vi "ziExample-Module-Scope.vi"() -> ()   [LabVIEW 2009]
doc: "Control a Zurich instrument device via the LabOne Labview API. \nRequirements: Zurich Instruments MFLI, HF2 or UHFLI \nThis example shows how to start a scope module and retrieve data.\n\n© Zurich Instruments AG, www.zhinst.com"
uses:
  <instrlib>/Zurich Instruments LabOne/Public/Modules/ziTypeModEnum.ctl
  <instrlib>/Zurich Instruments LabOne/Public/Configure/ziSetValueDouble.vi
  <instrlib>/Zurich Instruments LabOne/Public/Modules/ziModSetValueDoubleArray.vi
  <instrlib>/Zurich Instruments LabOne/Public/Configure/ziGetValueString.vi
  <instrlib>/Zurich Instruments LabOne/Public/Configure/ziSetValueDoubleArray.vi
  <instrlib>/Zurich Instruments LabOne/Public/Modules/ziModGetScopeWave.vi
  <instrlib>/Zurich Instruments LabOne/Public/Modules/ziModSetValueDouble.vi
  <instrlib>/Zurich Instruments LabOne/Zurich Instruments LabOne.lvlib
panel:
  in  "method":u16(ring)=1 items=["Exponential", "Uniform"]
  in  "length":i32=100 caption="Length (pts)"
  in  "segmentedcount":i32=100 caption="segmented count"
  in  "segmented":bool=TRUE
  out "?":sgl[][](graph)
  in  "mode":u16(ring)=1 items=["Time Domain"=1, "Freq Domain FFT"=3]
  in  "stop":bool
  in  "averagerweight":dbl=1.0 caption="averager/weight"
  out "?":cluster{dbl[], "Data Float":sgl[]}[](graph)
  out "Error Out":errorcluster
  in  "Address":string="DEV"
  out "Selected Device":string
  in  "subscribepath":string="scopes/0/wave" caption="Subscribe Path"
  # "Only for non-HF2"
  # "ziExample-Module-Scope.vi\nRequirements: HF2LI, UHFLI or MFLI\nsee block diagram for VI description"
  # "Tested Devices:\n- HF2LI\n- UHFLI\n- MFLI"
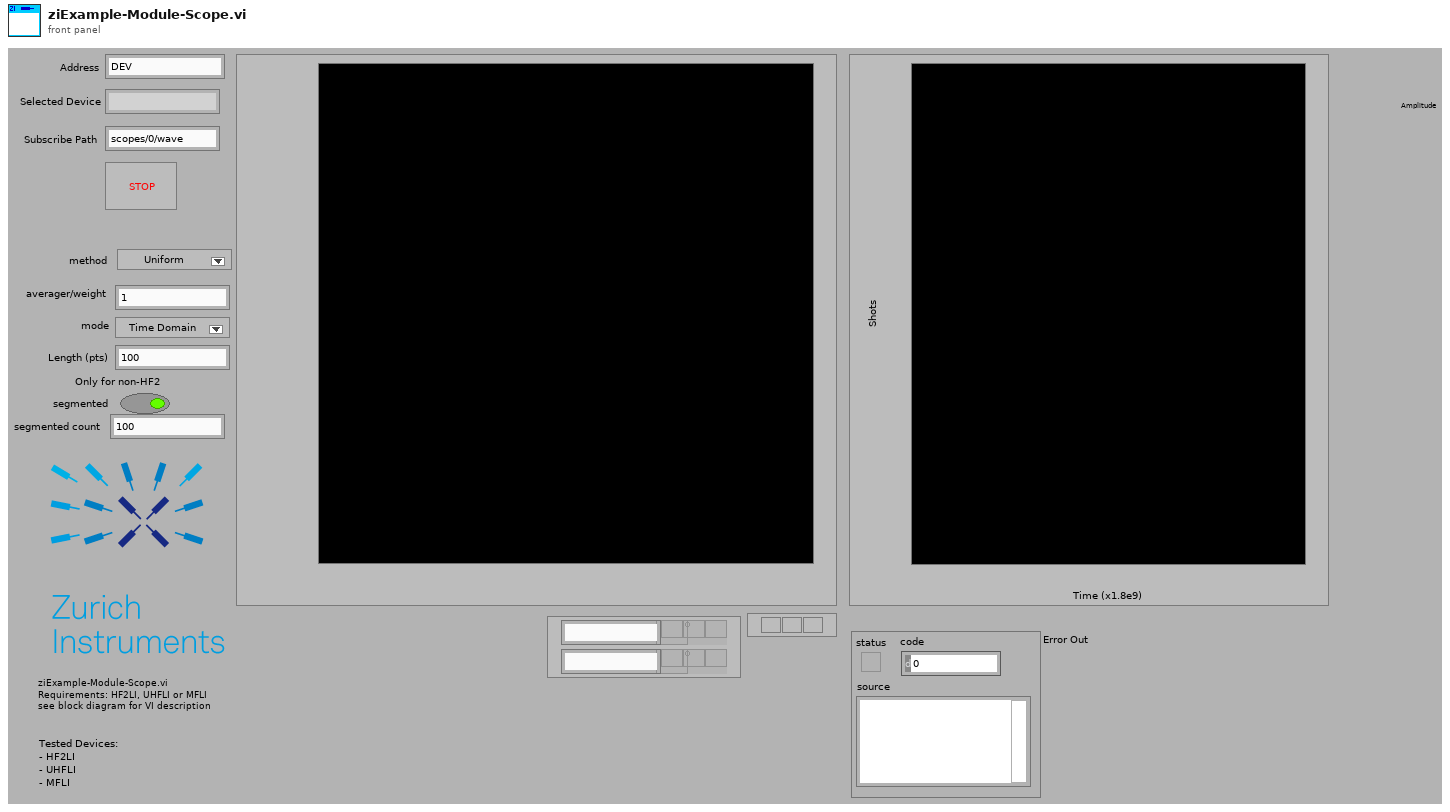
[diagram p1: front panel]
types:
  T1 = typedef "Zurich Instruments LabOne.lvlib/ziTypeModEnum.ctl" = u16
  T2 = typedef "Zurich Instruments LabOne.lvlib/ziTypeHandle.ctl" = cluster{"handleValid":bool, "Conn":u64, "Path Prefix":string, "Handle":u64, "Connected":bool, "Clockbase(s)":dbl}
  T3 = typedef "Zurich Instruments LabOne.lvlib/ziTypeModHandle.ctl" = cluster{"handleValid":bool, "Conn":u64, "ModHandle":u64, "moduleID":string, "Path Prefix":string}
  T4 = typedef "Zurich Instruments LabOne.lvlib/ziTypeModResults.ctl" = cluster{"PathArray":string[], "ValueType":T5, "NoOfResults":u64, "ziGenericHeader":T6[]}
  T5 = typedef "Zurich Instruments LabOne.lvlib/ziTypePollType.ctl" = enum16{"NONE", "DOUBLE_DATA", "INTEGER_DATA", "DEMOD_SAMPLE", "SCOPE_WAVE_HF2", "AUXIN_SAMPLE", "DIO_SAMPLE", "BYTE_ARRAY", "PWA_WAVE", "9", "10", "11", "12", "13", "14", "15", "TREE_CHANGE_DEPRI", "17", "ERROR", "19", "20", "21", "22", "23", "24", "25", "26", "27", "28", "29", "30", "31", "DOUBLE_DATA_TS", "INTEGER_DATA_TS", "34", "SCOPE_WAVE", "SCOPE_WAVE_EX", "37", "BYTE_ARRAY_TS", "39", "40", "41", "42", "43", "44", "45", "CNT_DATA", "47", "TREE_CHANGE", "49", "50", "51", "52", "53", "54", "55", "56", "57", "58", "59", "60", "61", "62", "63", "SWEEPER_DATA", "SPECTRUM_DATA", "ADVISOR_DATA", "VECTOR_DATA", "IMP_DATA", "SHF_GENERATOR_WAVEFORM_DATA", "SHF_RESULT_LOGGER_DATA", "SHF_SCOPE_DATA", "DEMOD_VECTOR"}
  T6 = typedef "Zurich Instruments LabOne.lvlib/ziTypeModGenericHeader.ctl" = cluster{"HeaderType":enum8{"HEADER_TYPE_NONE", "HEADER_TYPE_SWTRIGGER", "HEADER_TYPE_SWEEPER"}, "SampleFormat":u8, "SystemTime":timestamp, "CreatedTimeStamp":u64, "ChangedTimeStamp":u64, "Flags":u32, "ChunkSizeBytes":u64, "Name":string, "Status":u32, "GroupIndex":u32, "Color":u32, "ActiveRow":u32, "TriggerNumber":u64, "GridRows":u32, "GridCols":u32, "GridMode":u32, "GridOperation":u32, "GridDirection":u32, "GridRepetitions":u32, "GridColDelta":dbl, "GridColOffset":dbl, "GridRowDelta":dbl, "GridRowOffset":dbl, "Bandwidth":dbl, "Center":dbl, "Nenbw":dbl}
  T7 = typedef "Zurich Instruments LabOne.lvlib/ziTypeScopeWaveGrid.ctl" = cluster{"Timestamp (ticks)":u64, "Timestamp Trigger (ticks)":u64, "dt (s)":dbl, "Channel Enable":u8[], "Channel Input":enum8{"Signal Input 1", "Signal Input 2", "Trigger Input 1", "Trigger Input 2", "Aux Output 1", "Aux Output 2", "Aux Output 3", "Aux Output 4", "Aux Input 1", "Aux Input 2"}[], "Trigger Enable":u64, "Trigger Input":u64, "Channel BW Limit":u8[], "Channel Math":u8[], "Channel Scaling":sgl[], "Sequence Number":u32, "Segment Number":u32, "Block Number":u32, "Data Transfer Mode":enum8{"Single Transfer", "Block Transfer", "Continuous Transfer", "FFT Single Transfer"}, "Block Marker":enum8{"None", "End of Block"}, "Flags":u8, "Sample Format":enum8{"Int16", "Int32", "Float32", "reserved", "Int16 Interleaved", "Int32 Interleaved", "Float32 Interleaved"}, "Sample Count":u32, "Channel Offset":dbl[], "Data Int16":i16[][], "Data Int32":i32[][], "Data Float":sgl[][], "Total Samples":u32}
  T8 = typedef "Zurich Instruments LabOne.lvlib/ziTypeScopeWave.ctl" = cluster{"Timestamp (ticks)":u64, "Timestamp Trigger (ticks)":u64, "dt (s)":dbl, "Channel Enable":u8[], "Channel Input":enum8{"Signal Input 1", "Signal Input 2", "Trigger Input 1", "Trigger Input 2", "Aux Output 1", "Aux Output 2", "Aux Output 3", "Aux Output 4", "Aux Input 1", "Aux Input 2"}[], "Trigger Enable":u64, "Trigger Input":u64, "Channel BW Limit":u8[], "Channel Math":u8[], "Channel Scaling":sgl[], "Sequence Number":u32, "Segment Number":u32, "Block Number":u32, "Data Transfer Mode":enum8{"Single Transfer", "Block Transfer", "Continuous Transfer", "FFT Single Transfer"}, "Block Marker":enum8{"None", "End of Block"}, "Flags":u8, "Sample Format":enum8{"Int16", "Int32", "Float32", "reserved", "Int16 Interleaved", "Int32 Interleaved", "Float32 Interleaved"}, "Sample Count":u32, "Channel Offset":dbl[], "Data Int16":i16[], "Data Int32":i32[], "Data Float":sgl[], "Total Samples":u64}
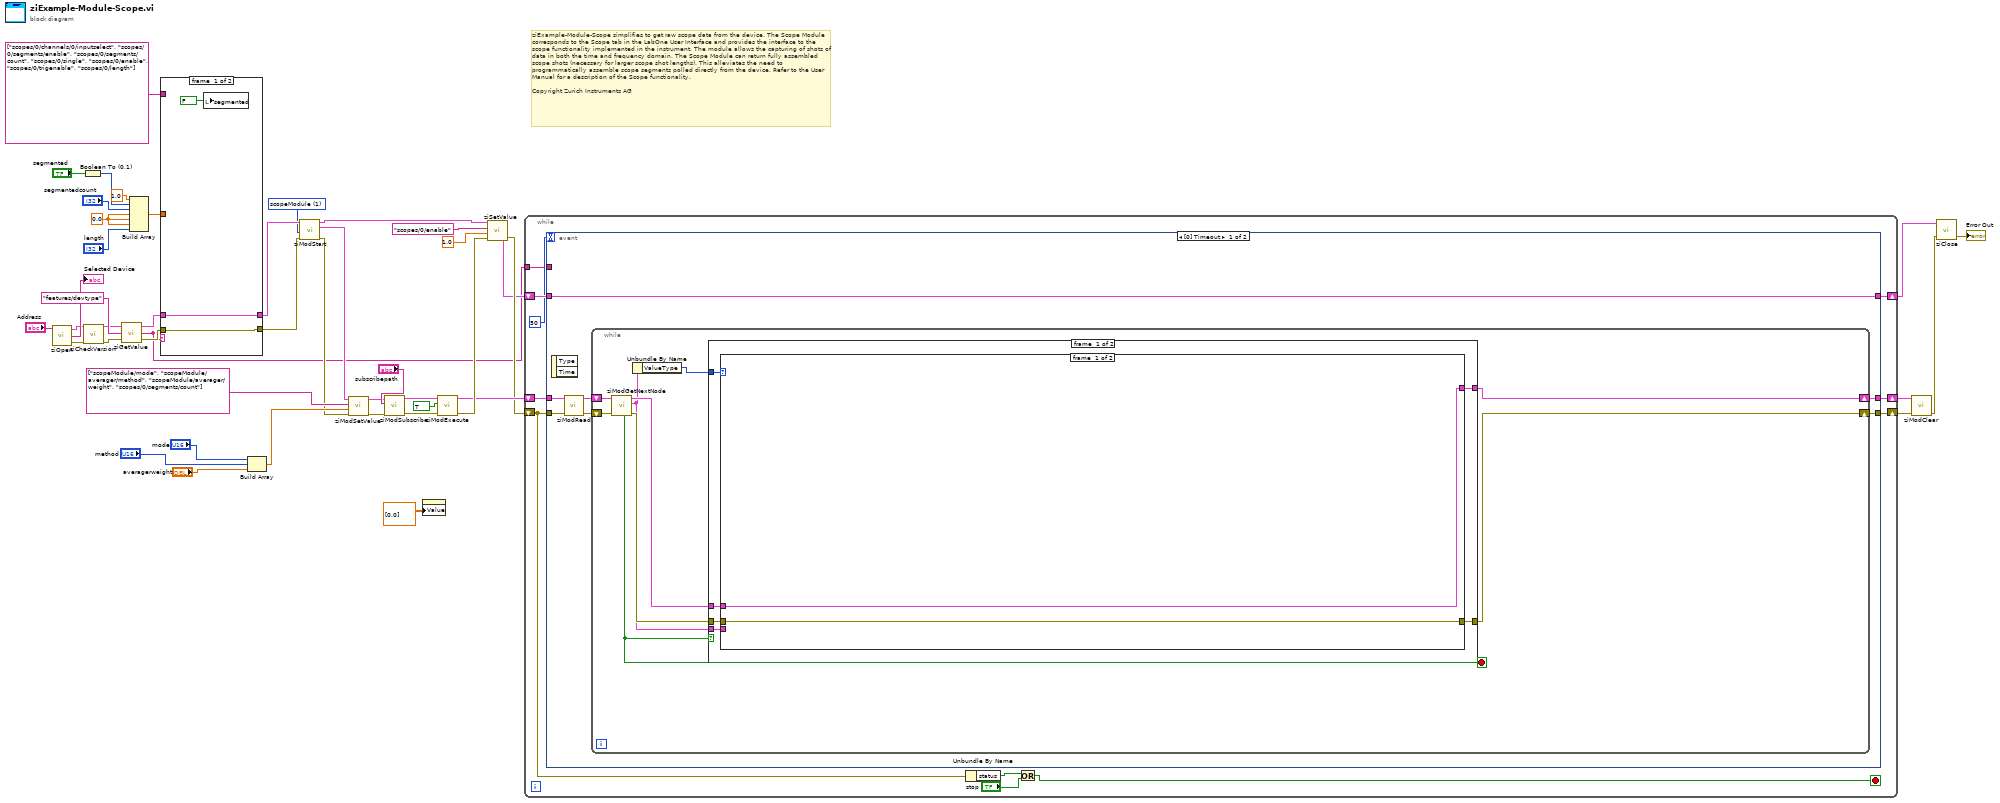
[diagram p0: block diagram]
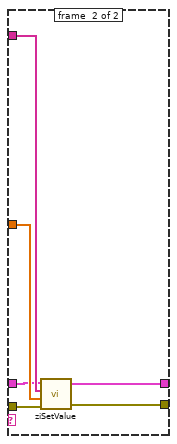
[diagram p2: hidden frame]
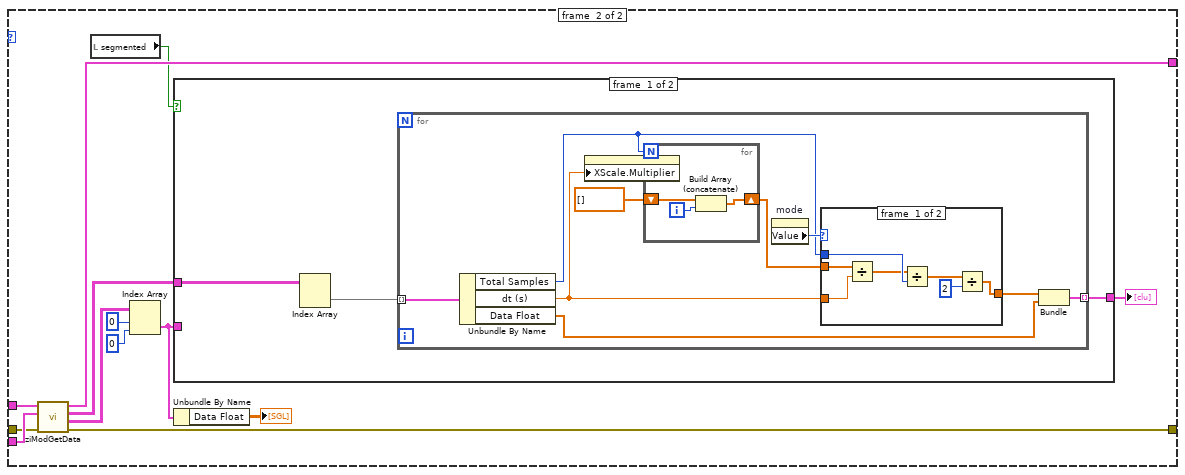
[diagram p3: hidden frame]
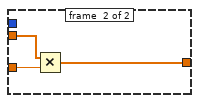
[diagram p4: hidden frame]
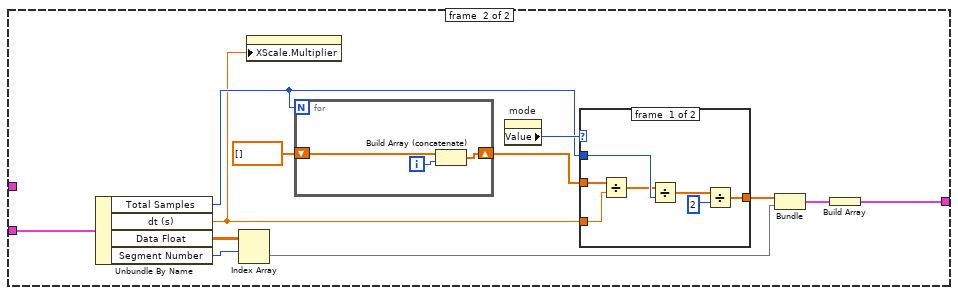
[diagram p5: hidden frame]
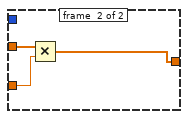
[diagram p6: hidden frame]
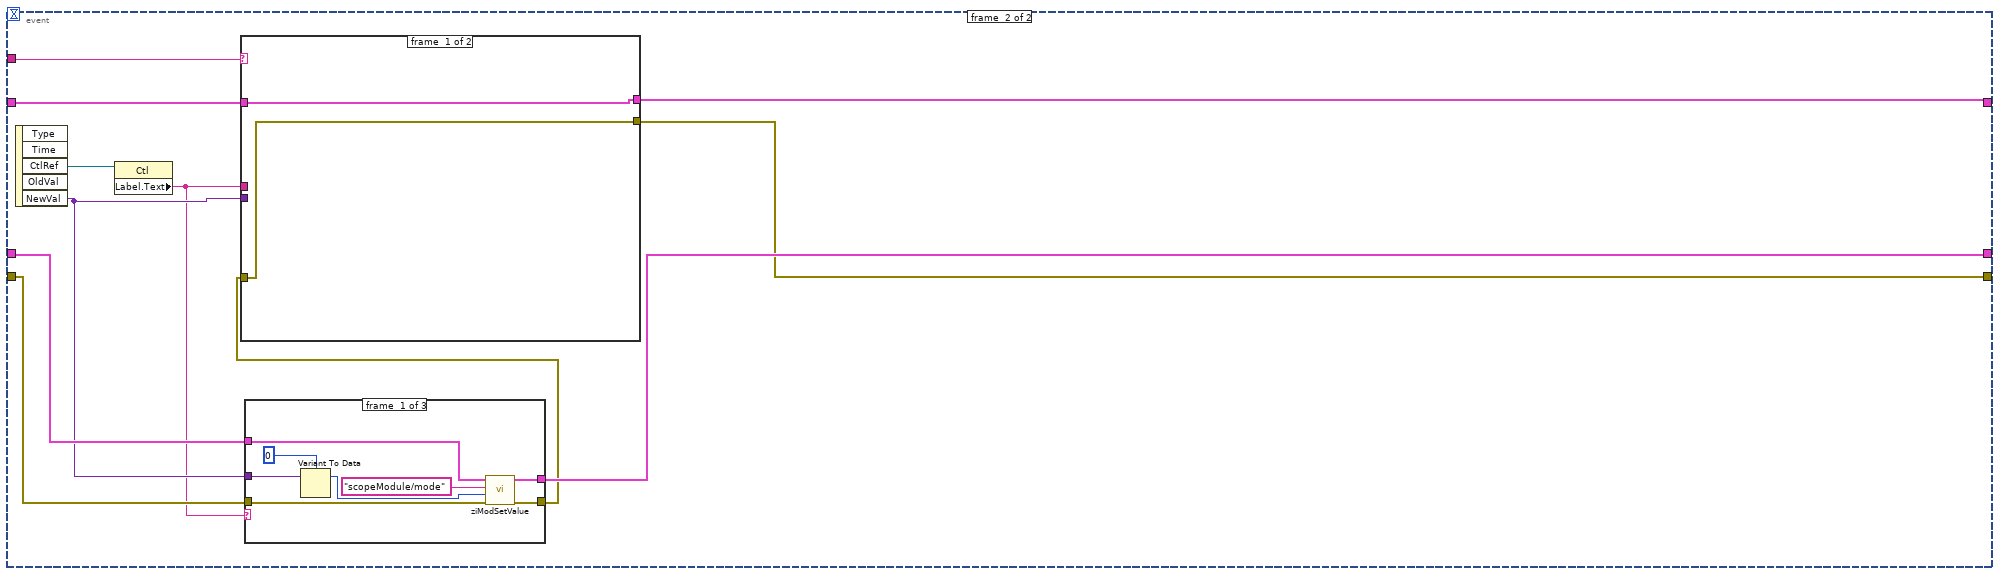
[diagram p8: hidden frame]
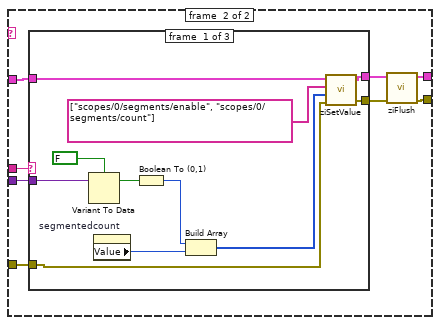
[diagram p9: hidden frame]
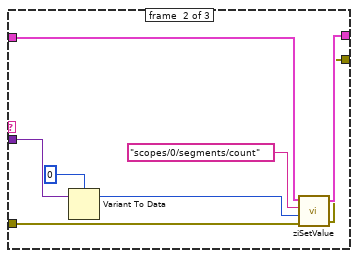
[diagram p10: hidden frame]
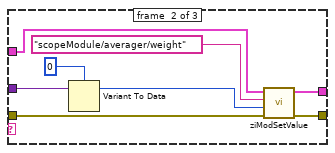
[diagram p12: hidden frame]
diagram:
  w5 = T1 1 items=["sweep", "scopeModule", "dataAcquisitionModule", "pidAdvisor", "awgModule", "impedanceModule", "multiDeviceSyncModule", "zoomFFT", "trigger", "deviceSettings", "record"] ("module Id")
  w11 = 0.0 ("element")
  # "ziExample-Module-Scope simplifies to get raw scope data from the device. The Scope Module corresponds to the Scope tab in the LabOne User Interface and provides the interface to the scope functionality implemented in the instrument. The module allows the capturing of shots of data in both the time and frequency domain. The Scope Module can return fully assembled scope shots (necessary for larger scope shot lengths). This alleviates the need to programmatically assemble scope segments polled directly from the device. Refer to the User Manual for a description of the Scope functionality.\n\nCopyright Zurich Instruments AG"
  n1 = call <instrlib>:"ziOpen.vi"("Address"="Address") -> ("Error Out"=w8:errorcluster, "Selected Device"=→"Selected Device":string, "HandleOut"=w9:T2)  [unwired: 1 in, 2 out]
  n2 = Boolean To (0,1)(Boolean="segmented") -> (0, 1=w25:i16)
  n3 = call <instrlib>:"ziCheckVersion.vi"("Handle In"=w9, "Error In"=w8) -> ("Handle Out"=w6:T2, "Error Out"=w7:errorcluster)  [unwired: 11 in, 1 out]
  n4 = call-poly <instrlib>:"ziGetValue.vi"("error in"=w7, "Path"="features/devtype", "Handle In"=w6) -> ("error out"=w14:errorcluster, "Value"=w13:string, "Handle Out"=w15:T2)
  n5 = Build Array(1.0 ("element"), w25, "segmentedcount", w11, w11, w11, "length") -> (w27:dbl[])
  n6 = case shown="\"HF2IS\", \"HF2LI\"" w13 {
    tunnel: [w49 w56] -> w45
    tunnel: string[] ["scopes/0/channels/0/inputselect", "scopes/0/segments/enable", "scopes/0/segments/count", "scopes/0/single", "scopes/0/enable", "scopes/0/trigenable", "scopes/0/length"] -> [_ w55]
    tunnel: [w50 w54] -> w32
    tunnel: w27 -> [_ w53]
    tunnel: w15 -> [w50 w52]
    tunnel: w14 -> [w49 w51]
    frame #0 {
      n7 = local write "segmented"(FALSE ("segmented")) -> ()
    }
    frame #1 {
      n8 = call-poly <instrlib>:"ziSetValue.vi"("Error In"=w51, "Values"=w53, "Paths"=w55, "Handle In"=w52) -> ("Error Out"=w56:errorcluster, "Handle Out"=w54:T2)  [unwired: 1 in]
    }
  }
  n9 = Build Array("mode", "method", "averagerweight") -> (w23:dbl[])
  n10 = call <instrlib>:"ziModStart.vi"("Error In"=w45, "module Id"=w5, "Handle In"=w32) -> ("Error Out"=w19:errorcluster, "ModHandle Out"=w20:T3, "Handle Out"=w12:T2)  [unwired: 6 in]
  n11 = call-poly <instrlib>:"ziModSetValue.vi"("Error In"=w19, "Values"=w23, "Paths"=string[] ["scopeModule/mode", "scopeModule/averager/method", "scopeModule/averager/weight", "scopes/0/segments/count"], "ModHandle In"=w20) -> ("Error Out"=w18:errorcluster, "ModHandle Out"=w17:T3)  [unwired: 6 in]
  n12 = call <instrlib>:"ziModSubscribe.vi"("Error In"=w18, "Path"="subscribepath", "ModHandle In"=w17) -> ("Error Out"=w37:errorcluster, "ModHandle Out"=w38:T3)  [unwired: 6 in]
  n13 = property class="IntGraph (strict)"("Value"=dbl[][] [[0.0]]) -> ()  [unwired: 2 in, 2 out]
  n14 = call <instrlib>:"ziModExecute.vi"("Error In"=w37, "Modal (F)"=TRUE ("Modal"), "ziModHandle In"=w38) -> ("Error Out"=w36:errorcluster, "ziModHandle Out"=w31:T3)  [unwired: 6 in]
  n15 = call-poly <instrlib>:"ziSetValue.vi"("Error In"=w36, "Value"=1.0, "Path"="scopes/0/enable", "Handle In"=w12) -> ("Error Out"=w30:errorcluster, "Handle Out"=w29:T2)  [unwired: 1 in]
  n16 = while {
    shift-right: [w66] -> w42
    shift-left: w30 -> [w57]
    shift-right: [w65] -> w41
    shift-left: w31 -> [w67]
    shift-right: [w63] -> w28
    shift-left: w29 -> [w64]
    tunnel: w13 -> [w61]
    stop <- w58 stop-if-true
    n17 = event shown="[0] Timeout" {
      selector: _ -> [_ _]
      dyn-events: _ -> [_ _]
      timeout: 50 -> [_ _]
      tunnel: w67 -> [w72 w165]
      tunnel: w57 -> [w71 w166]
      tunnel: [w70 w162] -> w66
      tunnel: [w69 w164] -> w65
      tunnel: w64 -> [w68 w161]
      tunnel: [w68 w163] -> w63
      tunnel: w61 -> [_ w157]
      event #0 {
        n18 = event-data() -> ()  [unwired: 1 in, 2 out]
        n19 = call <instrlib>:"ziModRead.vi"("error in"=w71, "ziModHandle In"=w72) -> ("error out"=w74:errorcluster, "ziModHandle Out"=w73:T3)  [unwired: 8 in]
        n20 = while {
          shift-right: [w82] -> w69
          shift-left: w73 -> [w76]
          shift-right: [w81] -> w70
          shift-left: w74 -> [w77]
          stop <- w75 stop-if-true
          n21 = call <instrlib>:"ziModGetNextNode.vi"("Error In"=w77, "ModHandle In"=w76) -> ("Error Out"=w80:errorcluster, "ModResults"=w78:T4, "ModHandle Out"=w83:T3, "NoData"=w75:bool)  [unwired: 6 in]
          n22 = Unbundle By Name(w78) -> ("ValueType"=w79:T5)
          n23 = case shown="False" w75 {
            tunnel: w83 -> [w89 w155]
            tunnel: [w88 w155] -> w82
            tunnel: [w87 w156] -> w81
            tunnel: w80 -> [w86 w156]
            tunnel: w78 -> [w85 _]
            tunnel: w79 -> [w84 _]
            frame #0 {
              n24 = case shown="\"SCOPE_WAVE_EX\"" w84 {
                tunnel: w89 -> [w91 w101]
                tunnel: w85 -> [_ w104]
                tunnel: w86 -> [w90 w103]
                tunnel: [w90 w102] -> w87
                tunnel: [w91 w100] -> w88
                frame #0 {
                }
                frame #1 {
                  n25 = call-poly <instrlib>:"ziModGetData.vi"("Error In"=w103, "ModResults"=w104, "ModHandle In"=w101) -> ("Error Out"=w102:errorcluster, "ModScopeWaveGrid"=w98:T7[][], "ModScopeWave"=w94:T8[][], "ModHandle Out"=w100:T3)  [unwired: 5 in]
                  n26 = local read "segmented"() -> (w93:bool)
                  n27 = Index Array(array=w98, index (row)=0, index (col)=0 ("disabled index (col)")) -> (element=w92:T7)
                  n28 = case shown="True" w93 {
                    tunnel: [w107 w132] -> w99
                    tunnel: w94 -> [w106 _]
                    tunnel: w92 -> [_ w141]
                    frame #0 {
                      n29 = Index Array(array=w106) -> (element=w105:T8[])  [unwired: 2 in]
                      n30 = for {
                        tunnel: w105 -> [w116] mode=indexing
                        tunnel: [w114] -> w107 mode=indexing
                        n31 = Unbundle By Name(w116) -> ("Total Samples"=w110:u64, "dt (s)"=w108:dbl, "Data Float"=w113:sgl[])
                        n32 = property class="IntGraph (strict)"("XScale.Multiplier"=w108) -> ()  [unwired: 2 in, 2 out]
                        n33 = for {
                          N: w110 -> [_]
                          shift-right: [w128] -> w111
                          shift-left: dbl[] [] -> [w129]
                          i -> [w127]
                          n34 = Build Array (concatenate)(w129, w127) -> (w128:dbl[])
                        }
                        n35 = property on="mode" class="Ring (strict)"() -> ("Value"=w112:u16)  [unwired: 2 in, 2 out]
                        n36 = case shown="1, Default" w112 {
                          tunnel: w108 -> [w123 w126]
                          tunnel: w111 -> [w122 w125]
                          tunnel: w110 -> [w121 _]
                          tunnel: [w117 w124] -> w109
                          frame #0 {
                            n37 = Divide(x=w122, y=w123) -> (x/y=w120:dbl[])
                            n38 = Divide(x=w120, y=w121) -> (x/y=w119:dbl[])
                            n39 = Divide(x=w119, y=2) -> (x/y=w117:dbl[])
                          }
                          frame #1 {
                            n40 = Multiply(x=w125, y=w126) -> (x*y=w124:dbl[])
                          }
                        }
                        n41 = Bundle(w109, "Data Float"=w113) -> (w114:cluster{dbl[], "Data Float":sgl[]})  [unwired: 1 in]
                      }
                    }
                    frame #1 {
                      n42 = Unbundle By Name(w141) -> ("Total Samples"=w137:u32, "dt (s)"=w135:dbl, "Data Float"=w131:sgl[][], "Segment Number"=w130:u32)
                      n43 = Index Array(array=w131, index (row)=w130) -> (element=w134:sgl[])  [unwired: 1 in]
                      n44 = property class="IntGraph (strict)"("XScale.Multiplier"=w135) -> ()  [unwired: 2 in, 2 out]
                      n45 = for {
                        N: w137 -> [_]
                        shift-right: [w153] -> w138
                        shift-left: dbl[] [] -> [w154]
                        i -> [w152]
                        n46 = Build Array (concatenate)(w154, w152) -> (w153:dbl[])
                      }
                      n47 = property on="mode" class="Ring (strict)"() -> ("Value"=w139:u16)  [unwired: 2 in, 2 out]
                      n48 = case shown="1, Default" w139 {
                        tunnel: w135 -> [w148 w151]
                        tunnel: w138 -> [w147 w150]
                        tunnel: w137 -> [w146 _]
                        tunnel: [w142 w149] -> w136
                        frame #0 {
                          n49 = Divide(x=w147, y=w148) -> (x/y=w145:dbl[])
                          n50 = Divide(x=w145, y=w146) -> (x/y=w144:dbl[])
                          n51 = Divide(x=w144, y=2) -> (x/y=w142:dbl[])
                        }
                        frame #1 {
                          n52 = Multiply(x=w150, y=w151) -> (x*y=w149:dbl[])
                        }
                      }
                      n53 = Bundle(w136, "Data Float"=w134) -> (w133:cluster{dbl[], "Data Float":sgl[]})  [unwired: 1 in]
                      n54 = Build Array(w133) -> (w132:cluster{dbl[], "Data Float":sgl[]}[])
                    }
                  }
                  "?" <- w99
                  n55 = Unbundle By Name(w92) -> ("Data Float"=→"?":sgl[][])
                }
              }
            }
            frame #1 {
            }
          }
        }
      }
      event #1 {
        n56 = event-data() -> ("CtlRef"=w167:refnum<vi>, "NewVal"=w159:variant)  [unwired: 1 in, 3 out]
        n57 = property class="Ctl"(reference=w167) -> ("Label.Text"=w158:string)  [unwired: 1 in, 2 out]
        n58 = case shown="\"mode\"" w158 {
          tunnel: w159 -> [w206 w214 _]
          tunnel: w166 -> [w203 w211 w216]
          tunnel: [w202 w210 w216] -> w160
          tunnel: w165 -> [w201 w209 w215]
          tunnel: [w200 w208 w215] -> w164
          frame #0 {
            n59 = Variant To Data(Variant=w206, type=u16 0) -> (data=w204:u16)  [unwired: 1 in, 1 out]
            n60 = call-poly <instrlib>:"ziModSetValue.vi"("Error In"=w203, "Value"=w204, "Path"="scopeModule/mode", "ModHandle In"=w201) -> ("Error Out"=w202:errorcluster, "ModHandle Out"=w200:T3)  [unwired: 6 in]
          }
          frame #1 {
            n61 = Variant To Data(Variant=w214, type=0) -> (data=w212:i32)  [unwired: 1 in, 1 out]
            n62 = call-poly <instrlib>:"ziModSetValue.vi"("Error In"=w211, "Value"=w212, "Path"="scopeModule/averager/weight", "ModHandle In"=w209) -> ("Error Out"=w210:errorcluster, "ModHandle Out"=w208:T3)  [unwired: 6 in]
          }
          frame #2 {
          }
        }
        n63 = case shown="Default" w157 {
          tunnel: [w168 w177] -> w163
          tunnel: [w169 w176] -> w162
          tunnel: w161 -> [w168 w174]
          tunnel: w160 -> [w169 w173]
          tunnel: w159 -> [_ w172]
          tunnel: w158 -> [_ w171]
          frame #0 {
          }
          frame #1 {
            n64 = case shown="\"segmented\"" w171 {
              tunnel: w172 -> [w188 w196 _]
              tunnel: w174 -> [w185 w193 w198]
              tunnel: [w184 w192 w198] -> w175
              tunnel: w173 -> [w183 w191 w197]
              tunnel: [w182 w190 w197] -> w170
              frame #0 {
                n65 = Variant To Data(Variant=w188, type=FALSE ("segmented 2")) -> (data=w186:bool)  [unwired: 1 in, 1 out]
                n66 = property on="segmentedcount" class="DigNum (strict)"() -> ("Value"=w178:i32)  [unwired: 2 in, 2 out]
                n67 = Boolean To (0,1)(Boolean=w186) -> (0, 1=w180:i16)
                n68 = Build Array(w180, w178) -> (w179:i32[])
                n69 = call-poly <instrlib>:"ziSetValue.vi"("Error In"=w183, "Values"=w179, "Paths"=string[] ["scopes/0/segments/enable", "scopes/0/segments/count"], "Handle In"=w185) -> ("Error Out"=w182:errorcluster, "Handle Out"=w184:T2)  [unwired: 1 in]
              }
              frame #1 {
                n70 = Variant To Data(Variant=w196, type=0) -> (data=w195:i32)  [unwired: 1 in, 1 out]
                n71 = call-poly <instrlib>:"ziSetValue.vi"("Error In"=w191, "Value"=w195, "Path"="scopes/0/segments/count", "Handle In"=w193) -> ("Error Out"=w190:errorcluster, "Handle Out"=w192:T2)  [unwired: 1 in]
              }
              frame #2 {
              }
            }
            n72 = call <instrlib>:"ziFlush.vi"("error in"=w170, "Handle In"=w175) -> ("error out"=w176:errorcluster, "Handle Out"=w177:T2)  [unwired: 8 in]
          }
        }
      }
    }
    n73 = Unbundle By Name(w57) -> ("status"=w60:bool)
    n74 = Or(x=w60, y="stop") -> (x .or. y?=w58:bool)
  }
  n75 = call <instrlib>:"ziModClear.vi"("Error In"=w42, "ziModHandle In"=w41) -> ("Error Out"=w47:errorcluster)  [unwired: 7 in, 1 out]
  n76 = call <instrlib>:"ziClose.vi"("Error In"=w47, "Handle In"=w28) -> ("Error Out"=→"Error Out":errorcluster)  [unwired: 2 in, 1 out]
